vi "initialize runtime configuration by implementation.vi"(8 "error in (no error)":errorcluster, 10 "Runtime Implementation":T1, 11 "E2E configuration in":refnum<class "E2E Tag Exchange configuration.lvclass">) -> (0 "error out":errorcluster, 2 "Runtime Specific Configuration":variant, 3 "E2E configuration out":refnum<class "E2E Tag Exchange configuration.lvclass">)   [LabVIEW 2015, in "E2E Tag Exchange configuration.lvclass"]
uses:
  E2E Tag Exchange configuration.lvclass
  Runtime Implementation.ctl
  E2E Tag Exchange configuration.lvclass/E2E Tag Exchange configuration.ctl
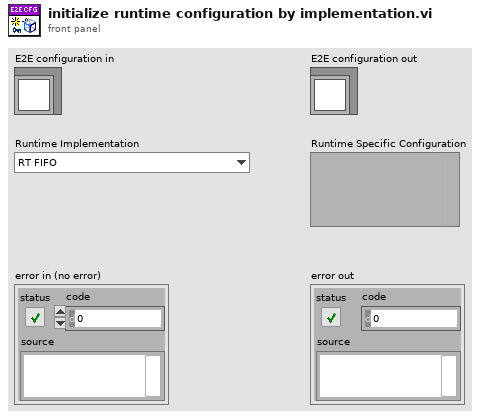
[diagram p1: front panel]
types:
  T1 = typedef "E2E Tag Exchange configuration.lvclass/Runtime Implementation.ctl" = enum16{"RT FIFO", "UDP"}
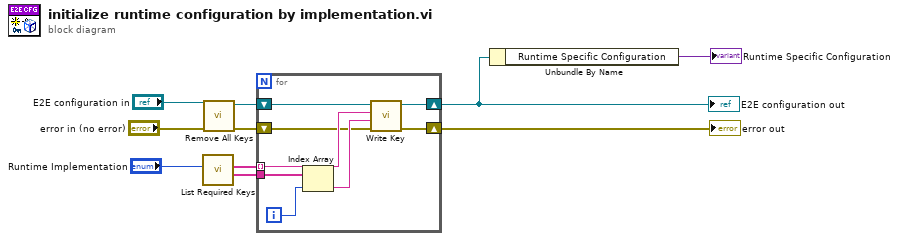
[diagram p0: block diagram]
diagram:
  n1 = call "List Required Keys.vi"("Runtime Implementation"="Runtime Implementation") -> ("Initial Values"=w5:string[], "Requested Keys"=w4:string[])  [unwired: 9 in]
  n2 = call "Remove All Keys.vi"("error in"="error in (no error)", "E2E configuration in"="E2E configuration in") -> ("error out"=w6:errorcluster, "E2E configuration out"=w7:refnum<class "E2E Tag Exchange configuration.lvclass">)  [unwired: 8 in]
  n3 = for {
    tunnel: w4 -> [w15] mode=indexing
    tunnel: w5 -> [w18]
    shift-right: [w11] -> w3
    shift-left: w7 -> [w16]
    shift-right: [w12] -> w2
    shift-left: w6 -> [w13]
    i -> [w17]
    n4 = Index Array(array=w18, index=w17) -> (element=w14:string)
    n5 = call "Write Key.vi"("error in"=w13, "Value"=w14, "Key"=w15, "E2E configuration in"=w16) -> ("error out"=w12:errorcluster, "E2E configuration out"=w11:refnum<class "E2E Tag Exchange configuration.lvclass">)  [unwired: 6 in]
  }
  "E2E configuration out" <- w3
  "error out" <- w2
  n6 = Unbundle By Name(w3) -> ("Runtime Specific Configuration"=→"Runtime Specific Configuration":variant)
